vi "Load Default Configuration.vi"(8 "error in (no error)":errorcluster, 10 "Default Configuration":variant, 11 "CIFTemplateNode in":refnum<class "CIFTemplateNode.lvclass">) -> (0 "error out":errorcluster, 3 "CIFTemplateNode out":refnum<class "CIFTemplateNode.lvclass">)   [LabVIEW 2021, in "CIFTemplateNode.lvclass"]
uses:
  CIFTemplateNode.lvclass
  CIFTemplateNode.lvclass/CIFTemplateNode.ctl
  CIFTemplateCoreOOB/OOB_Rx/CIFTemplateCoreOOB_Rx.lvclass
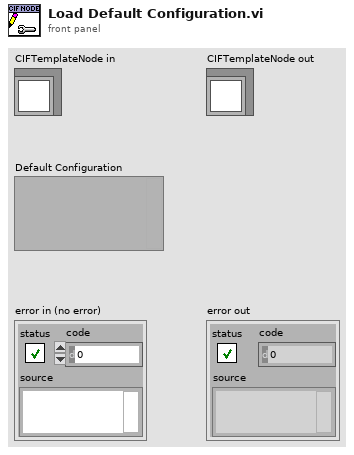
[diagram p1: front panel]
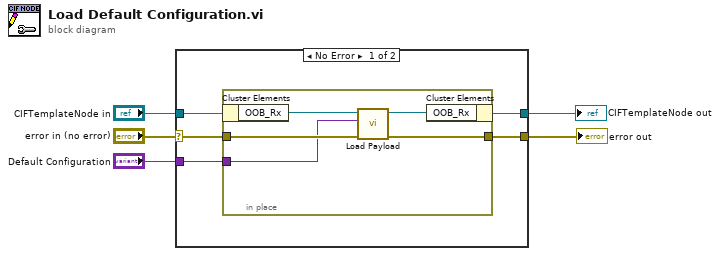
[diagram p0: block diagram]
diagram:
  n1 = case shown="No Error" "error in (no error)" {
    selector: "error in (no error)" -> [w9 w16]
    tunnel: [w8 w16] -> w4
    tunnel: [w7 w17] -> w2
    tunnel: "CIFTemplateNode in" -> [w10 w17]
    tunnel: "Default Configuration" -> [w6 _]
    frame No Error {
      n2 = in-place {
        in-place-border: w9 -> [w13]
        in-place-border: [w12] -> w8
        in-place-border: w6 -> [w11]
        n3 = in-place-cluster #1(w10) -> ("OOB_Rx"=w15:refnum<class "CIFTemplateCoreOOB_Rx.lvclass">)
        n4 = call "Load Payload.vi"("error in (no error)"=w13, "Configuration Payload"=w11, "CoreOOB_Rx in"=w15) -> ("error out"=w12:errorcluster, "CoreOOB_Rx out"=w14:refnum<class "CIFTemplateCoreOOB_Rx.lvclass">)  [unwired: 7 in]
        n5 = in-place-cluster #1("OOB_Rx"=w14) -> (w7:refnum<class "CIFTemplateNode.lvclass">)
      }
    }
    frame Error {
    }
  }
  "error out" <- w4
  "CIFTemplateNode out" <- w2
